vi "Grayscale RGB Overlay.vi"(5 "Crop ROI?":bool, 7 "Grayscale Edge Image":T1, 8 "error in (no error)":errorcluster, 9 "RGB ROI Mask Image":T1, 10 "Depth History":refnum<queue>, 11 "RGB Frame Image In":T1) -> (0 "error out":errorcluster, 1 "Standard Dev":dbl, 2 "Average Depth":dbl, 3 "RGB ROI Image Out":T1, 4 "Filtered Depth Values":dbl[](array[numeric]))   [LabVIEW 2018]
uses:
  <vilib>/vision/Image Controls.llb/IMAQ Image.ctl
  <vilib>/vision/NI_Vision_Development_Module.lvlib
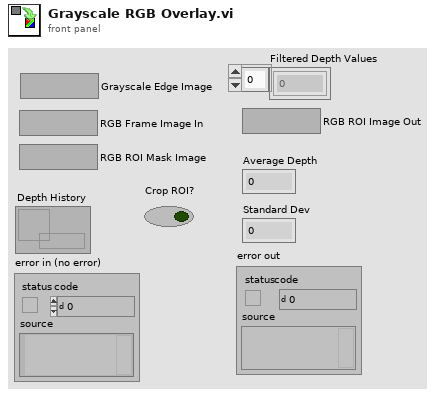
[diagram p1: front panel]
types:
  T1 = typedef "IMAQ Image.ctl" = refnum<image>
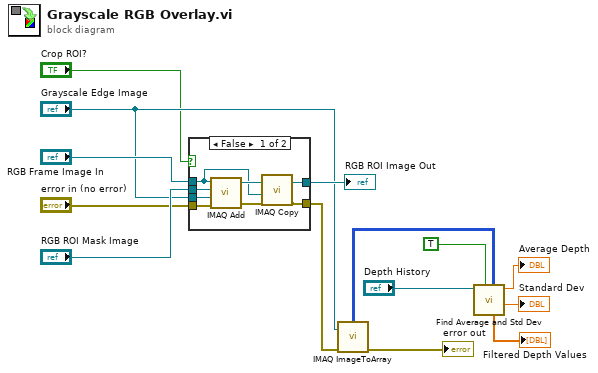
[diagram p0: block diagram]
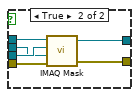
[diagram p2: hidden frame]
diagram:
  n1 = case shown="False" "Crop ROI?" {
    tunnel: "RGB Frame Image In" -> [w16 w27]
    tunnel: [w19 w23] -> w8
    tunnel: "RGB ROI Mask Image" -> [w22 w25]
    tunnel: "error in (no error)" -> [w21 w28]
    tunnel: [w18 w24] -> w4
    tunnel: "Grayscale Edge Image" -> [w20 w26]
    frame False {
      n2 = call "IMAQ Add"("Image Src A"=w16, "Image Dst"=w22, "Image Src B"=w20, "error in (no error)"=w21) -> ("Image Dst Out"=w17:T1, "error out"=w15:errorcluster)  [unwired: 3 in]
      n3 = call "IMAQ Copy"("error in (no error)"=w15, "Image Dst"=w16, "Image Src"=w17) -> ("error out"=w19:errorcluster, "Image Dst Out"=w18:T1)  [unwired: 3 in]
    }
    frame True {
      n4 = call "IMAQ Mask"("error in (no error)"=w28, "Image Dst"=w25, "Image Mask"=w26, "Image Src"=w27) -> ("error out"=w23:errorcluster, "Image Dst Out"=w24:T1)  [unwired: 1 in]
    }
  }
  "RGB ROI Image Out" <- w4
  n5 = call "IMAQ ImageToArray"("error in (no error)"=w8, "Image"="Grayscale Edge Image") -> ("error out"=→"error out":errorcluster, "Image Pixels (U8)"=w14:u8[][])  [unwired: 2 in, 3 out]
  n6 = call "Find Average and Std Dev.vi"("ROI"=w14, "Use ROI?"=TRUE, "Depth History"="Depth History") -> ("Std Dev."=→"Standard Dev":dbl, "Average Depth"=→"Average Depth":dbl, "Filtered Depth Values"=→"Filtered Depth Values":dbl[])  [unwired: 6 in]
